vi "rad_Target Configuration Options Dialog.vi"(8 "error in":errorcluster, 11 "Target Configuration Options":T1={"NumInBatch"=0, "Target Config Operation"=enum."No Config", "Target Name"="", "Increment Static IPs"=FALSE, "Change Target Name"=FALSE, "Primary NIC"={"MAC address"="", "IP Address Request Mode"=2, "IP address"="", "Subnet mask"="", "Gateway"="", "DNS server"=""}} {"Primary NIC"."IP Address Request Mode" items=["Static"=1, "DHCP/Link-Local"=2, "Link-Local Only"=4, "DHCP Only"=8]}) -> (0 "error out":errorcluster, 1 "Cancelled":bool, 3 "Target Configuration Options":T1={"NumInBatch"=0, "Target Config Operation"=enum."No Config", "Target Name"="", "Increment Static IPs"=FALSE, "Change Target Name"=FALSE, "Primary NIC"={"MAC address"="", "IP Address Request Mode"=2, "IP address"="", "Subnet mask"="", "Gateway"="", "DNS server"=""}} {"Primary NIC"."IP Address Request Mode" items=["Static"=1, "DHCP/Link-Local"=2, "Link-Local Only"=4, "DHCP Only"=8]})   [LabVIEW 2013]
uses:
  TypeDefs/rad_Target Configuration Settings.ctl
  TypeDefs/rad_Target Configuration Operations.ctl
  Targets/TypeDefs/rad_Target Network Settings.ctl
  Util/FP Control/FP Control Functions.ctl
panel:
  in  "State Variables":cluster{"Target Configuration Options":T1}={"Target Configuration Options"={"NumInBatch"=0, "Target Config Operation"=enum."No Config", "Target Name"="", "Increment Static IPs"=FALSE, "Change Target Name"=FALSE, "Primary NIC"={"MAC address"="", "IP Address Request Mode"=2, "IP address"="", "Subnet mask"="", "Gateway"="", "DNS server"=""}}} {"Target Configuration Options"."Primary NIC"."IP Address Request Mode" items=["Static"=1, "DHCP/Link-Local"=2, "Link-Local Only"=4, "DHCP Only"=8]}
  in  "Restore Defaults":bool
  in  "SetAsDefault":bool
  in  "Change Target Name":bool
  in  "Increment IP":bool
  in  "Deployment Batch Size":u32=1 min=1 max=100
  in  "IP Address Request Mode":i32(ring)=2 items=["Static"=1, "DHCP/Link-Local"=2, "Link-Local Only"=4, "DHCP Only"=8]
  in  "DNS":string
  in  "Gateway":string
  in  "Subnet Mask":string
  in  "IP Address":string
  in  "Target Name (no spaces)":string="RTController"
  in  "Cancel":bool
  in  "OK":bool
  in  "Primary NIC Settings":enum32{"Existing", "Image", "Specify"}(radio)
  # "Batch Image Deployment"
  # "Network Configuration"
  # "Secondary NIC Settings"
  # "RAD deployment always applies the network configuration\nfound in the image to all secondary NICs on the target."
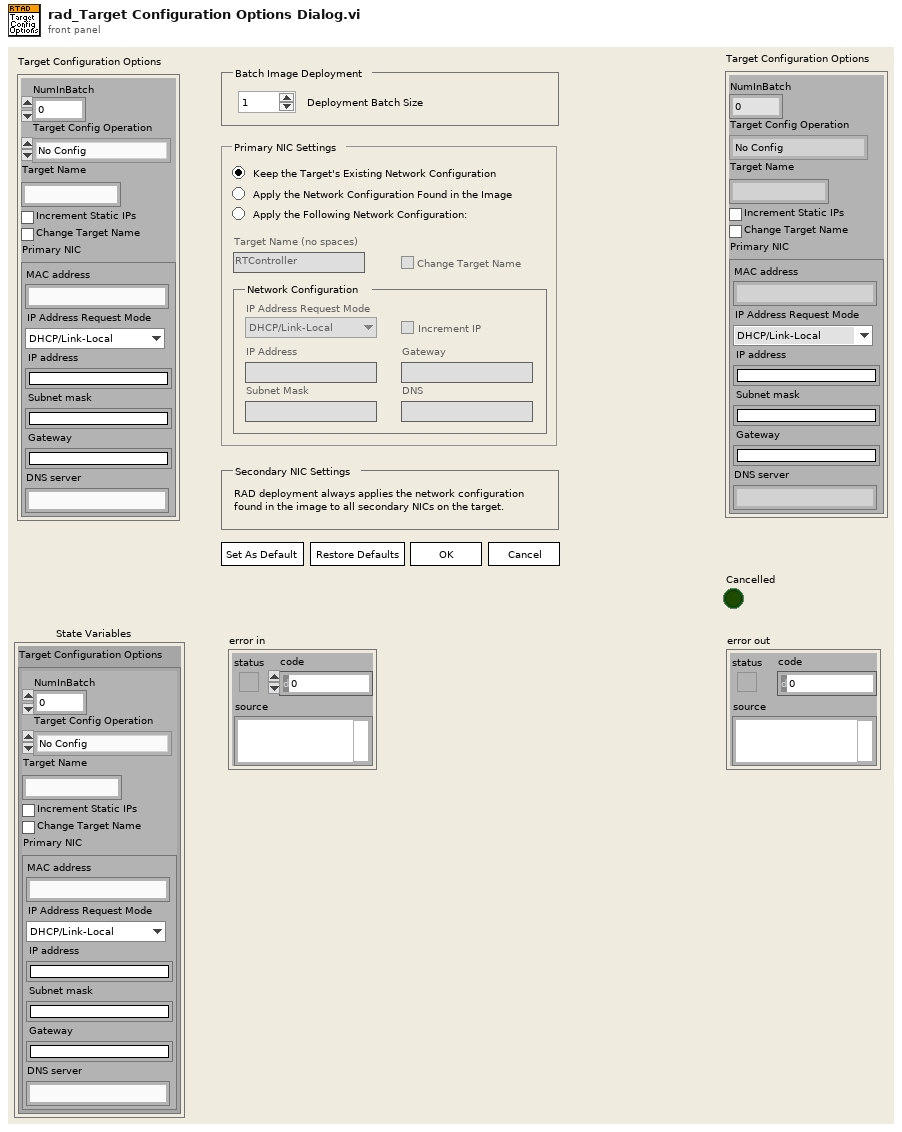
[diagram p1: front panel]
types:
  T1 = typedef "rad_Target Configuration Settings.ctl" = cluster{"NumInBatch":u32, "Target Config Operation":T2, "Target Name":string, "Increment Static IPs":bool, "Change Target Name":bool, "Primary NIC":T3}
  T2 = typedef "rad_Target Configuration Operations.ctl" = enum8{"No Config", "Image Config", "Static Config"}
  T3 = typedef "rad_Target Network Settings.ctl" = cluster{"MAC address":string, "IP Address Request Mode":i32, "IP address":string, "Subnet mask":string, "Gateway":string, "DNS server":string}
  T4 = typedef "FP Control Functions.ctl" = enum16{"Open", "Close", "Bring To Front", "Center"}
  T5 = enum8{"Enabled", "Disabled", "Disabled and Grayed Out"}
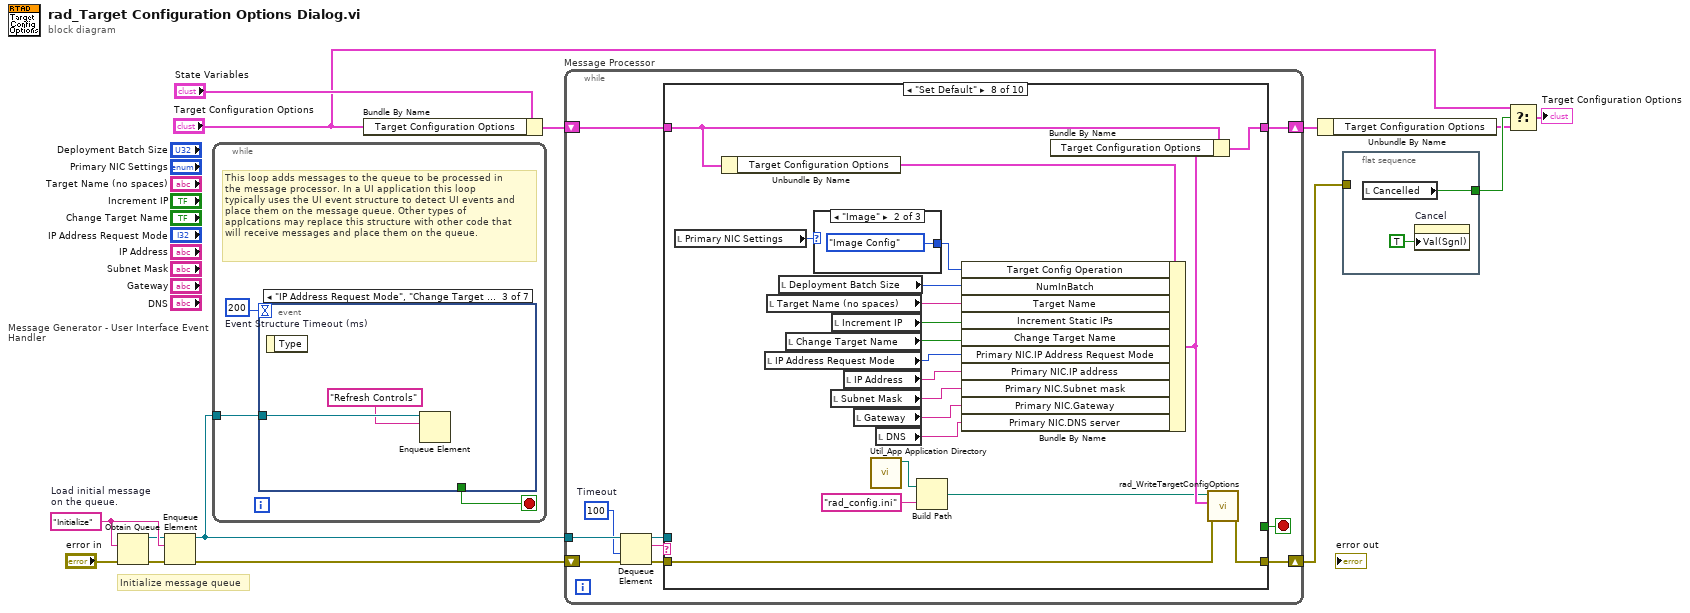
[diagram p0: block diagram]
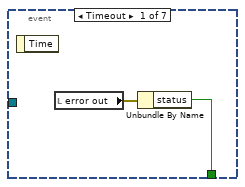
[diagram p2: hidden frame]
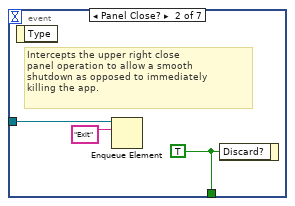
[diagram p3: hidden frame]
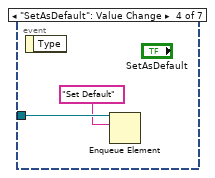
[diagram p4: hidden frame]
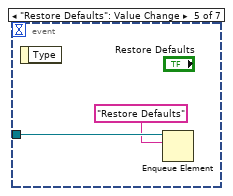
[diagram p5: hidden frame]
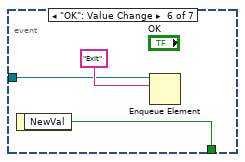
[diagram p6: hidden frame]
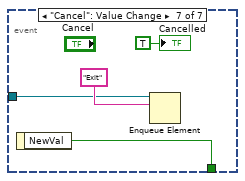
[diagram p7: hidden frame]
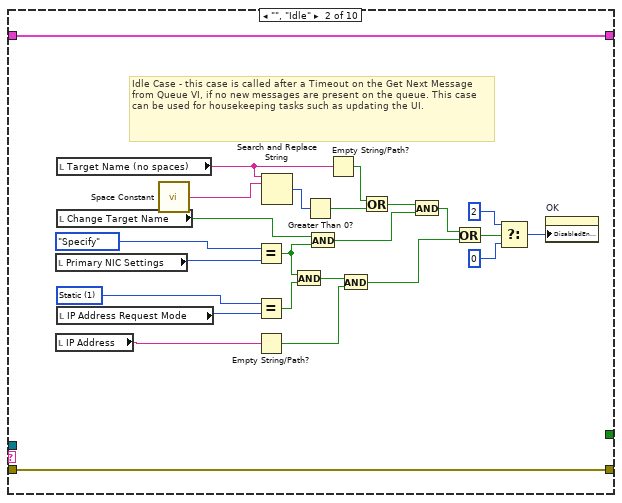
[diagram p9: hidden frame]
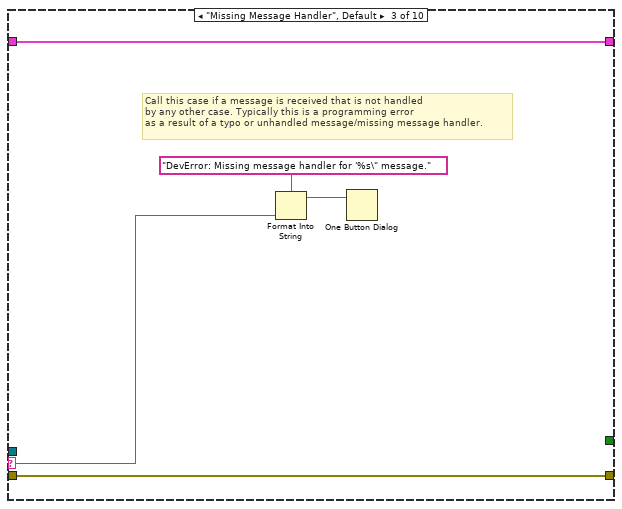
[diagram p10: hidden frame]
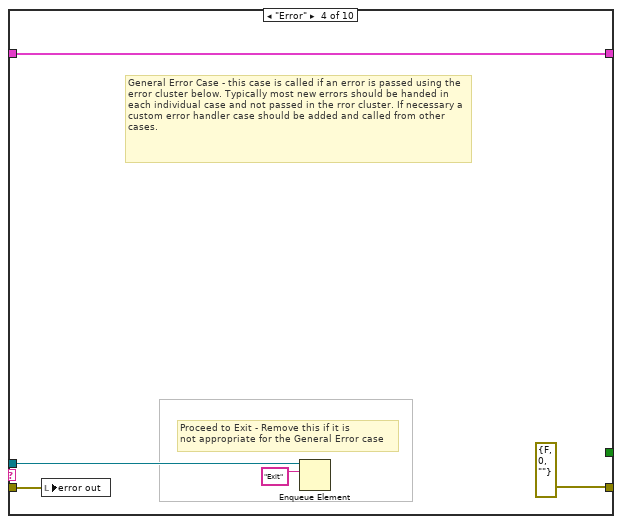
[diagram p11: hidden frame]
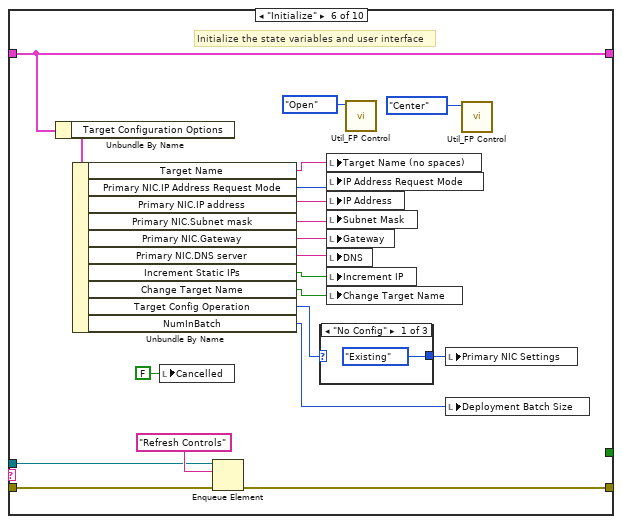
[diagram p13: hidden frame]
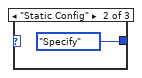
[diagram p14: hidden frame]
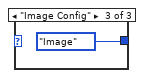
[diagram p15: hidden frame]
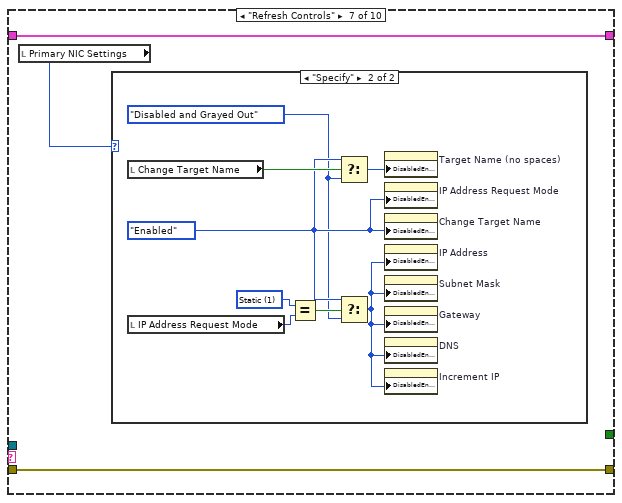
[diagram p16: hidden frame]
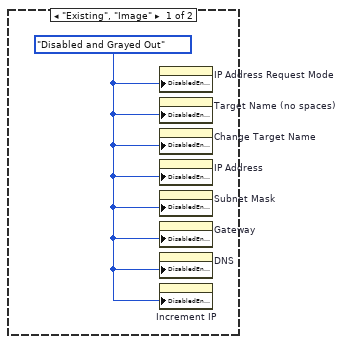
[diagram p17: hidden frame]
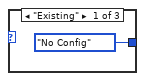
[diagram p18: hidden frame]
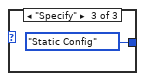
[diagram p19: hidden frame]
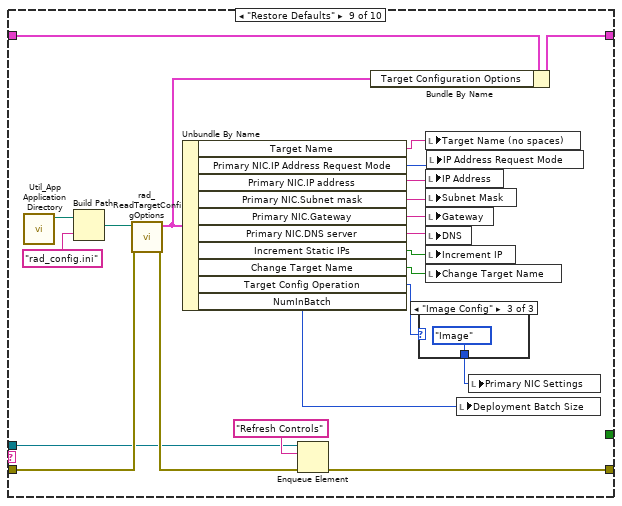
[diagram p20: hidden frame]
diagram:
  w3 = "Initialize"  # Load initial message on the queue.
  # "Initialize message queue"
  n1 = Obtain Queue(element data type=w3, error in (no error)="error in") -> (queue out=w1:refnum<queue>, error out=w14:errorcluster)  [unwired: 3 in, 1 out]
  n2 = Enqueue Element(queue=w1, element=w3, error in (no error)=w14) -> (queue out=w2:refnum<queue>, error out=w4:errorcluster)  [unwired: 1 in, 1 out]
  n3 = while "Message Generator - User Interface Event Handler" {
    tunnel: w2 -> [w15]
    stop <- w16 stop-if-true
    w17 = 200  # Event Structure Timeout (ms)
    # "This loop adds messages to the queue to be processed in\nthe message processor. In a UI application this loop\ntypically uses the UI event structure to detect UI events and\nplace them on the message queue. Other types of\napplcations may replace this structure with other code that\nwill receive messages and place them on the queue."
    n4 = event shown="[2] \"IP Address Request Mode\", \"Change Target Name\", \"Primary NIC Settings\": Value Change" {
      selector: _ -> [_ _ _ _ _ _ _]
      dyn-events: _ -> [_ _ _ _ _ _ _]
      timeout: w17 -> [_ _ _ _ _ _ _]
      tunnel: [w18 w22 _ _ _ w29 w33] -> w16
      tunnel: w15 -> [_ w20 w24 w26 w28 w30 w34]
      event Timeout {
        n5 = event-data() -> ()  [unwired: 2 out]
        n6 = local read "error out"() -> (w19:errorcluster)
        n7 = Unbundle By Name(w19) -> ("status"=w18:bool)
      }
      event Panel Close? {
        w22 = TRUE ("Discard?")
        # "Intercepts the upper right close\npanel operation to allow a smooth\nshutdown as opposed to immediately\nkilling the app."
        n8 = event-data() -> ()  [unwired: 2 out]
        n9 = Enqueue Element(queue=w20, element="Exit") -> ()  [unwired: 2 in, 3 out]
        n10 = event-data("Discard?"=w22) -> ()  [unwired: 1 in, 1 out]
      }
      event "IP Address Request Mode", "Change Target Name", "Primary NIC Settings": Value Change {
        n11 = event-data() -> ()  [unwired: 2 out]
        n12 = Enqueue Element(queue=w24, element="Refresh Controls") -> ()  [unwired: 2 in, 3 out]
      }
      event "SetAsDefault": Value Change {
        n13 = event-data() -> ()  [unwired: 2 out]
        n14 = Enqueue Element(queue=w26, element="Set Default") -> ()  [unwired: 2 in, 3 out]
      }
      event "Restore Defaults": Value Change {
        n15 = event-data() -> ()  [unwired: 2 out]
        n16 = Enqueue Element(queue=w28, element="Restore Defaults") -> ()  [unwired: 2 in, 3 out]
      }
      event "OK": Value Change {
        n17 = event-data() -> ("NewVal"=w29:bool)  [unwired: 1 out]
        n18 = Enqueue Element(queue=w30, element="Exit") -> ()  [unwired: 2 in, 3 out]
      }
      event "Cancel": Value Change {
        n19 = event-data() -> ("NewVal"=w33:bool)  [unwired: 1 out]
        n20 = Enqueue Element(queue=w34, element="Exit") -> ()  [unwired: 2 in, 3 out]
        "Cancelled" <- TRUE ("Cancelled")
      }
    }
  }
  n21 = Bundle By Name(cluster="State Variables", "Target Configuration Options"="Target Configuration Options") -> (w12:cluster{"Target Configuration Options":T1})
  n22 = while "Message Processor" {
    shift-left: w4 -> [w41]
    shift-right: [w43] -> w9
    tunnel: w2 -> [w37]
    shift-left: w12 -> [w45]
    shift-right: [w44] -> w10
    stop <- w38 stop-if-true
    w36 = 100  # Timeout
    n23 = Dequeue Element(queue=w37, timeout in ms (-1)=w36, error in (no error)=w41) -> (queue out=w42:refnum<queue>, element=w39:string, error out=w40:errorcluster)  [unwired: 1 out]
    n24 = case shown="\"Set Default\"" w39 {
      selector: w39 -> [_ _ w75 _ _ _ _ _ _ _]
      tunnel: [w47 w72 w77 w82 w84 w96 w110 w137 w151 w170] -> w44
      tunnel: w45 -> [w47 w72 w77 w82 w84 w96 w110 w138 w153 w171]
      tunnel: w42 -> [_ _ _ w80 _ w93 _ _ w145 w186]
      tunnel: w40 -> [w46 w71 w76 w78 w83 w92 w109 w131 w149 w187]
      tunnel: [w46 w71 w76 errorcluster {"status"=FALSE, "code"=0, "source"=""} ("error out") w83 w91 w109 w130 w147 w185] -> w43
      tunnel: [_ _ _ _ _ _ _ _ _ TRUE] -> w38
      frame "---------- Framework Operations ----------" {
        # "Dummy case to add a seperator in the Case Structure menu"
      }
      frame "", "Idle" {
        w49 = 1 items=["Static"=1, "DHCP/Link-Local"=2, "Link-Local Only"=4, "DHCP Only"=8] ("IP Address Request Mode")
        # "Idle Case - this case is called after a Timeout on the Get Next Message from Queue VI, if no new messages are present on the queue. This case can be used for housekeeping tasks such as updating the UI."
        n25 = local read "Primary NIC Settings"() -> (w58:enum32{"Existing", "Image", "Specify"})
        n26 = local read "IP Address"() -> (w68:string)
        n27 = local read "Target Name (no spaces)"() -> (w57:string)
        n28 = local read "Change Target Name"() -> (w53:bool)
        n29 = local read "IP Address Request Mode"() -> (w50:i32)
        n30 = call <vilib>:"Space Constant.vi"() -> ("String"=w70:string)
        n31 = Equal?(x=enum32{"Existing", "Image", "Specify"}."Specify" ("NIC Source"), y=w58) -> (x = y?=w52:bool)
        n32 = Equal?(x=w49, y=w50) -> (x = y?=w48:bool)
        n33 = Empty String/Path?(string/path=w68) -> (empty?=w67:bool)
        n34 = Search and Replace String(input string=w57, search string=w70) -> (number of replacements=w69:i32)  [unwired: 6 in, 3 out]
        n35 = And(x=w52, y=w48) -> (x .and. y?=w66:bool)
        n36 = Greater Than 0?(x=w69) -> (x > 0?=w55:bool)
        n37 = And(x=w53, y=w52) -> (x .and. y?=w51:bool)
        n38 = Empty String/Path?(string/path=w57) -> (empty?=w56:bool)
        n39 = And(x=w66, y=w67) -> (x .and. y?=w64:bool)
        n40 = Or(x=w56, y=w55) -> (x .or. y?=w54:bool)
        n41 = And(x=w54, y=w51) -> (x .and. y?=w65:bool)
        n42 = Or(x=w65, y=w64) -> (x .or. y?=w63:bool)
        n43 = Select(t=2, s=w63, f=0) -> (s? t:f=w60:i32)
        n44 = property on="OK" class="Bool"("DisabledEnum"=w60) -> ()  [unwired: 2 in, 2 out]
      }
      frame "Missing Message Handler", Default {
        # "Call this case if a message is received that is not handled \nby any other case. Typically this is a programming error\nas a result of a typo or unhandled message/missing message handler."
        n45 = Format Into String(format string="DevError: Missing message handler for '%s\" message." ("message"), w75) -> (resulting string=w73:string)  [unwired: 2 in, 1 out]
        n46 = One Button Dialog(message=w73) -> ()  [unwired: 2 out]
      }
      frame "Error" {
        # "Proceed to Exit - Remove this if it is\nnot appropriate for the General Error case"
        # "General Error Case - this case is called if an error is passed using the error cluster below. Typically most new errors should be handed in each individual case and not passed in the rror cluster. If necessary a custom error handler case should be added and called from other cases."
        n47 = local write "error out"(w78) -> ()
        n48 = Enqueue Element(queue=w80, element="Exit") -> ()  [unwired: 2 in, 3 out]
      }
      frame "---------- Generic Operations ----------" {
        # "Dummy case to add a seperator in the Case Structure menu"
      }
      frame "Initialize" {
        # "Initialize the state variables and user interface"
        n49 = Unbundle By Name(w96) -> ("Target Configuration Options"=w95:T1)
        n50 = Unbundle By Name(w95) -> ("Target Name"=w103:string, "Primary NIC.IP Address Request Mode"=w104:i32, "Primary NIC.IP address"=w102:string, "Primary NIC.Subnet mask"=w101:string, "Primary NIC.Gateway"=w100:string, "Primary NIC.DNS server"=w99:string, "Increment Static IPs"=w98:bool, "Change Target Name"=w97:bool, "Target Config Operation"=w90:T2, "NumInBatch"=w86:u32)
        n51 = local write "Cancelled"(FALSE ("Cancelled")) -> ()
        n52 = Enqueue Element(queue=w93, element="Refresh Controls", error in (no error)=w92) -> (error out=w91:errorcluster)  [unwired: 1 in, 2 out]
        n53 = case shown="\"No Config\"" w90 {
          tunnel: [enum32{"Existing", "Image", "Specify"}."Existing" ("NIC Source") enum32{"Existing", "Image", "Specify"}."Specify" ("NIC Source") enum32{"Existing", "Image", "Specify"}."Image" ("NIC Source")] -> w85
          frame "No Config" {
          }
          frame "Static Config" {
          }
          frame "Image Config" {
          }
        }
        n54 = local write "Target Name (no spaces)"(w103) -> ()
        n55 = local write "IP Address Request Mode"(w104) -> ()
        n56 = local write "IP Address"(w102) -> ()
        n57 = local write "Subnet Mask"(w101) -> ()
        n58 = local write "Gateway"(w100) -> ()
        n59 = local write "DNS"(w99) -> ()
        n60 = local write "Increment IP"(w98) -> ()
        n61 = local write "Change Target Name"(w97) -> ()
        n62 = call "Util_FP Control.vi"("Function"=FP_Control_Functions."Open") -> ()  [unwired: 10 in, 1 out]
        n63 = local write "Primary NIC Settings"(w85) -> ()
        n64 = local write "Deployment Batch Size"(w86) -> ()
        n65 = call "Util_FP Control.vi"("Function"=FP_Control_Functions."Center") -> ()  [unwired: 10 in, 1 out]
      }
      frame "Refresh Controls" {
        n66 = local read "Primary NIC Settings"() -> (w108:enum32{"Existing", "Image", "Specify"})
        n67 = case shown="\"Specify\"" w108 {
          frame "Existing", "Image" {
            w111 = T5."Disabled and Grayed Out" ("Disabled")
            n68 = property on="IP Address Request Mode" class="Ring (strict)"("DisabledEnum"=w111) -> ()  [unwired: 2 in, 2 out]
            n69 = property on="Target Name (no spaces)" class="Str"("DisabledEnum"=w111) -> ()  [unwired: 2 in, 2 out]
            n70 = property on="Change Target Name" class="Bool (strict)"("DisabledEnum"=w111) -> ()  [unwired: 2 in, 2 out]
            n71 = property on="IP Address" class="Str"("DisabledEnum"=w111) -> ()  [unwired: 2 in, 2 out]
            n72 = property on="Subnet Mask" class="Str"("DisabledEnum"=w111) -> ()  [unwired: 2 in, 2 out]
            n73 = property on="Gateway" class="Str"("DisabledEnum"=w111) -> ()  [unwired: 2 in, 2 out]
            n74 = property on="DNS" class="Str"("DisabledEnum"=w111) -> ()  [unwired: 2 in, 2 out]
            n75 = property on="Increment IP" class="Bool (strict)"("DisabledEnum"=w111) -> ()  [unwired: 2 in, 2 out]
          }
          frame "Specify" {
            w116 = 1 items=["Static"=1, "DHCP/Link-Local"=2, "Link-Local Only"=4, "DHCP Only"=8] ("IP Address Request Mode")
            w112 = T5."Disabled and Grayed Out" ("Disabled")
            w113 = T5."Enabled" ("Disabled")
            n76 = local read "Change Target Name"() -> (w118:bool)
            n77 = local read "IP Address Request Mode"() -> (w115:i32)
            n78 = Equal?(x=w116, y=w115) -> (x = y?=w114:bool)
            n79 = Select(t=w113, s=w118, f=w112) -> (s? t:f=w117:T5)
            n80 = Select(t=w113, s=w114, f=w112) -> (s? t:f=w119:T5)
            n81 = property on="Target Name (no spaces)" class="Str"("DisabledEnum"=w117) -> ()  [unwired: 2 in, 2 out]
            n82 = property on="IP Address Request Mode" class="Ring (strict)"("DisabledEnum"=w113) -> ()  [unwired: 2 in, 2 out]
            n83 = property on="Change Target Name" class="Bool (strict)"("DisabledEnum"=w113) -> ()  [unwired: 2 in, 2 out]
            n84 = property on="IP Address" class="Str"("DisabledEnum"=w119) -> ()  [unwired: 2 in, 2 out]
            n85 = property on="Subnet Mask" class="Str"("DisabledEnum"=w119) -> ()  [unwired: 2 in, 2 out]
            n86 = property on="Gateway" class="Str"("DisabledEnum"=w119) -> ()  [unwired: 2 in, 2 out]
            n87 = property on="DNS" class="Str"("DisabledEnum"=w119) -> ()  [unwired: 2 in, 2 out]
            n88 = property on="Increment IP" class="Bool (strict)"("DisabledEnum"=w119) -> ()  [unwired: 2 in, 2 out]
          }
        }
      }
      frame "Set Default" {
        n89 = local read "Primary NIC Settings"() -> (w139:enum32{"Existing", "Image", "Specify"})
        n90 = Unbundle By Name(w138) -> ("Target Configuration Options"=w136:T1)
        n91 = local read "IP Address Request Mode"() -> (w120:i32)
        n92 = local read "Target Name (no spaces)"() -> (w133:string)
        n93 = local read "Deployment Batch Size"() -> (w125:u32)
        n94 = local read "Change Target Name"() -> (w134:bool)
        n95 = case shown="\"Image\"" w139 {
          tunnel: [rad_Target_Configuration_Operations."No Config" ("Target Config Operation") rad_Target_Configuration_Operations."Image Config" ("Target Config Operation") rad_Target_Configuration_Operations."Static Config" ("Target Config Operation")] -> w126
          frame "Existing" {
          }
          frame "Image" {
          }
          frame "Specify" {
          }
        }
        n96 = local read "Subnet Mask"() -> (w122:string)
        n97 = local read "Increment IP"() -> (w135:bool)
        n98 = local read "IP Address"() -> (w121:string)
        n99 = local read "Gateway"() -> (w123:string)
        n100 = call "Util_App Application Directory.vi"() -> ("Application Directory"=w128:path)  [unwired: 11 out]
        n101 = local read "DNS"() -> (w124:string)
        n102 = Build Path(base path=w128, name or relative path="rad_config.ini" ("Config File Name")) -> (appended path=w127:path)
        n103 = Bundle By Name(cluster=w136, "Target Config Operation"=w126, "NumInBatch"=w125, "Target Name"=w133, "Increment Static IPs"=w135, "Change Target Name"=w134, "Primary NIC.IP Address Request Mode"=w120, "Primary NIC.IP address"=w121, "Primary NIC.Subnet mask"=w122, "Primary NIC.Gateway"=w123, "Primary NIC.DNS server"=w124) -> (w132:T1)
        n104 = Bundle By Name(cluster=w138, "Target Configuration Options"=w132) -> (w137:cluster{"Target Configuration Options":T1})
        n105 = call "rad_WriteTargetConfigOptions.vi"("error in (no error)"=w131, "TargetConfigurationOptions"=w132, "configuration file path"=w127) -> ("error out"=w130:errorcluster)  [unwired: 8 in]
      }
      frame "Restore Defaults" {
        n106 = call "Util_App Application Directory.vi"() -> ("Application Directory"=w154:path)  [unwired: 11 out]
        n107 = Build Path(base path=w154, name or relative path="rad_config.ini" ("Config File Name")) -> (appended path=w150:path)
        n108 = call "rad_ReadTargetConfigOptions.vi"("error in (no error)"=w149, "configuration file path"=w150) -> ("error out"=w148:errorcluster, "TargetConfigurationOptions"=w152:T1)  [unwired: 8 in]
        n109 = Unbundle By Name(w152) -> ("Target Name"=w163:string, "Primary NIC.IP Address Request Mode"=w164:i32, "Primary NIC.IP address"=w162:string, "Primary NIC.Subnet mask"=w161:string, "Primary NIC.Gateway"=w160:string, "Primary NIC.DNS server"=w159:string, "Increment Static IPs"=w158:bool, "Change Target Name"=w157:bool, "Target Config Operation"=w156:T2, "NumInBatch"=w144:u32)
        n110 = Enqueue Element(queue=w145, element="Refresh Controls", error in (no error)=w148) -> (error out=w147:errorcluster)  [unwired: 1 in, 2 out]
        n111 = Bundle By Name(cluster=w153, "Target Configuration Options"=w152) -> (w151:cluster{"Target Configuration Options":T1})
        n112 = case shown="\"Image Config\"" w156 {
          tunnel: [enum32{"Existing", "Image", "Specify"}."Existing" ("NIC Source") enum32{"Existing", "Image", "Specify"}."Specify" ("NIC Source") enum32{"Existing", "Image", "Specify"}."Image" ("NIC Source")] -> w143
          frame "No Config" {
          }
          frame "Static Config" {
          }
          frame "Image Config" {
          }
        }
        n113 = local write "Target Name (no spaces)"(w163) -> ()
        n114 = local write "IP Address"(w162) -> ()
        n115 = local write "Subnet Mask"(w161) -> ()
        n116 = local write "Gateway"(w160) -> ()
        n117 = local write "DNS"(w159) -> ()
        n118 = local write "Increment IP"(w158) -> ()
        n119 = local write "Change Target Name"(w157) -> ()
        n120 = local write "IP Address Request Mode"(w164) -> ()
        n121 = local write "Deployment Batch Size"(w144) -> ()
        n122 = local write "Primary NIC Settings"(w143) -> ()
      }
      frame "Exit" {
        # "Stop the VI\n>> Perform any cleanup tasks in this message case.\n>> Clear display before closing."
        n123 = local read "Primary NIC Settings"() -> (w173:enum32{"Existing", "Image", "Specify"})
        n124 = Release Queue(queue=w186, error in (no error)=w187) -> (error out=w185:errorcluster)  [unwired: 1 in, 2 out]
        n125 = local read "Deployment Batch Size"() -> (w175:u32)
        n126 = local read "IP Address Request Mode"() -> (w179:i32)
        n127 = local read "Target Name (no spaces)"() -> (w176:string)
        n128 = Unbundle By Name(w171) -> ("Target Configuration Options"=w172:T1)
        n129 = local read "Change Target Name"() -> (w178:bool)
        n130 = case shown="\"Existing\"" w173 {
          tunnel: [rad_Target_Configuration_Operations."No Config" ("Target Config Operation") rad_Target_Configuration_Operations."Image Config" ("Target Config Operation") rad_Target_Configuration_Operations."Static Config" ("Target Config Operation")] -> w174
          frame "Existing" {
          }
          frame "Image" {
          }
          frame "Specify" {
          }
        }
        n131 = local read "Subnet Mask"() -> (w181:string)
        n132 = local read "Increment IP"() -> (w177:bool)
        n133 = call "Util_FP Control.vi"("Function"=FP_Control_Functions."Close") -> ()  [unwired: 10 in, 1 out]
        n134 = local read "IP Address"() -> (w180:string)
        n135 = local read "Gateway"() -> (w182:string)
        n136 = local read "DNS"() -> (w183:string)
        n137 = Bundle By Name(cluster=w172, "NumInBatch"=w175, "Target Config Operation"=w174, "Target Name"=w176, "Increment Static IPs"=w177, "Change Target Name"=w178, "Primary NIC.IP Address Request Mode"=w179, "Primary NIC.IP address"=w180, "Primary NIC.Subnet mask"=w181, "Primary NIC.Gateway"=w182, "Primary NIC.DNS server"=w183) -> (w169:T1)
        n138 = Bundle By Name(cluster=w171, "Target Configuration Options"=w169) -> (w170:cluster{"Target Configuration Options":T1})
      }
    }
  }
  n139 = Unbundle By Name(w10) -> ("Target Configuration Options"=w7:T1)
  n140 = flat-sequence {
    tunnel: w9 -> [_]
    tunnel: [w192] -> w8
    frame #0 {
      n141 = local read "Cancelled"() -> (w192:bool)
      n142 = property on="Cancel" class="Bool"("Val(Sgnl)"=TRUE) -> ()  [unwired: 2 in, 2 out]
    }
  }
  n143 = Select(t="Target Configuration Options", s=w8, f=w7) -> (s? t:f=→"Target Configuration Options":T1)
